vi "Data2Array.vi"(4 "date":dbl) -> (1 "Array":dbl[](array[numeric]))   [LabVIEW 2014]
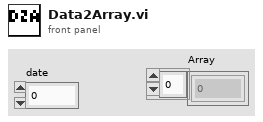
[diagram p1: front panel]
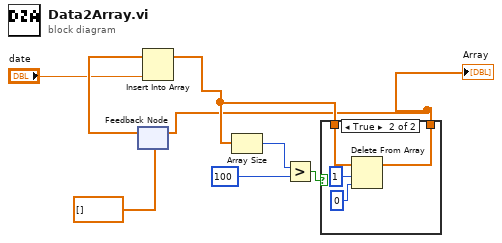
[diagram p0: block diagram]
diagram:
  n1 = feedback #1(dbl[] []) -> (w8:dbl[])
  n2 = Insert Into Array(array=w8, new element="date") -> (w3:dbl[])  [unwired: 1 in]
  n3 = Array Size(array=w3) -> (size(s)=w6:i32)
  n4 = Greater?(x=w6, y=100) -> (0:w4:bool)
  n5 = case shown="True" w4 {
    tunnel: w3 -> [w9 w13]
    tunnel: [w9 w12] -> w1
    frame False {
    }
    frame True {
      n6 = Delete From Array(array=w13, length=1, index=0) -> (array with subset deleted=w12:dbl[])  [unwired: 1 out]
    }
  }
  "Array" <- w1
  n7 = feedback-in #1(w1) -> ()
